vi "Waveform Test.vi"() -> (0 "error out":errorcluster, 1 "Result":bool, 2 "FileIds":string[](array[string]))   [LabVIEW 2018, in "Attach Test Files.lvlib"]
uses:
  <vilib>/Skyline/File/File/Send File.vi
  Attach Test Files.lvlib
  <vilib>/Skyline/File/File/NI Skyline File.lvclass
panel:
  out "Measured Data":dynamicdata(graph)
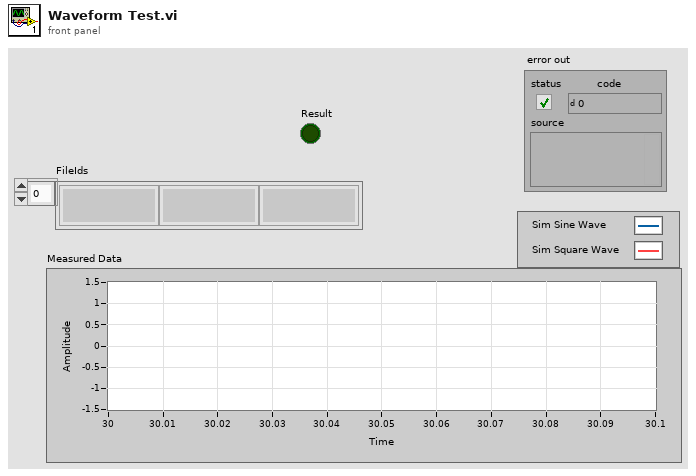
[diagram p1: front panel]
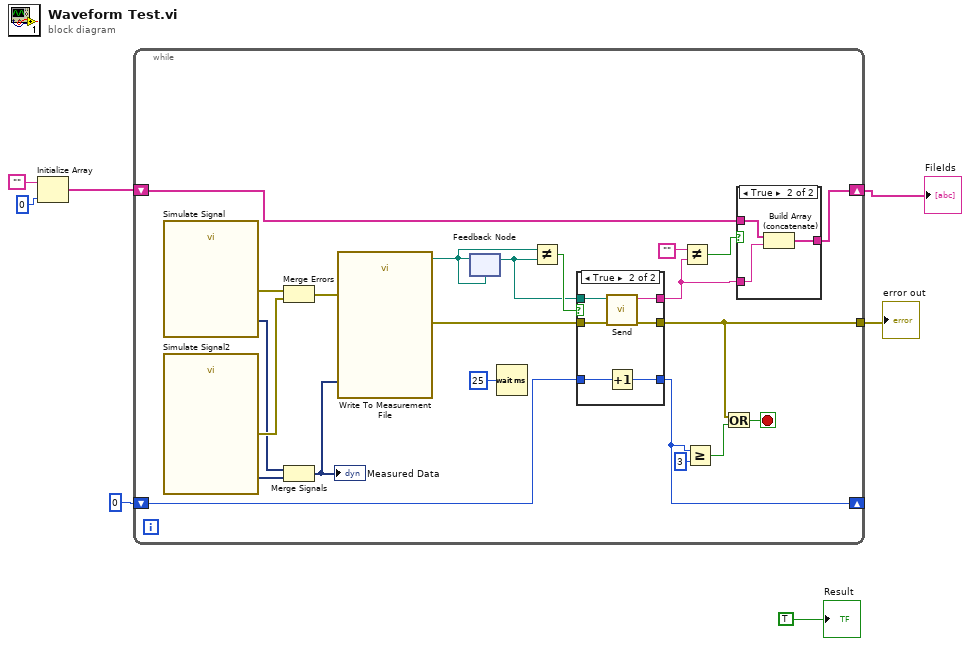
[diagram p0: block diagram]
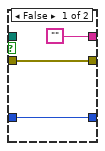
[diagram p3: hidden frame]
diagram:
  n1 = Initialize Array("", 0) -> (w4:string[])
  n2 = while {
    tunnel: [w20] -> w1
    shift-right: [w15] -> _
    shift-left: 0 -> [w16]
    shift-right: [w8] -> w2
    shift-left: w4 -> [w9]
    stop <- w24 stop-if-true
    n3 = call "Simulate Signal"() -> ("Sim Sine Wave"=w27:dynamicdata, "error out"=w29:errorcluster)  [unwired: 14 in]
    n4 = call "Simulate Signal2"() -> ("Sim Square Wave"=w26:dynamicdata, "error out"=w28:errorcluster)  [unwired: 14 in]
    n5 = Merge Errors(w29, w28) -> (w25:errorcluster)
    n6 = Merge Signals(w27, w26) -> (w22:dynamicdata)
    "Measured Data" <- w22
    n7 = call "Write To Measurement File"("Signals"=w22, "error in (no error)"=w25) -> ("Filename Out"=w17:path, "error out"=w18:errorcluster)  [unwired: 15 in, 1 out]
    n8 = feedback-in #1(w17) -> ()
    n9 = feedback #1(w17) -> (w19:path)
    n10 = Wait (ms)(milliseconds to wait=u32 25) -> ()  [unwired: 1 out]
    n11 = Not Equal?(x=w17, y=w19) -> (x != y?=w21:bool)
    n12 = case shown="True" w21 {
      tunnel: [w36 w41] -> w20
      tunnel: w19 -> [_ w40]
      tunnel: w18 -> [w36 w42]
      tunnel: w16 -> [w35 w39]
      tunnel: [w35 w38] -> w15
      tunnel: ["" w37] -> w10
      frame False {
      }
      frame True {
        n13 = call-poly <vilib>:"Send.vi"("error in (no error)"=w42, "path"=w40) -> ("error out"=w41:errorcluster, "id"=w37:string)  [unwired: 7 in]
        n14 = Increment(x=w39) -> (x+1=w38:i32)
      }
    }
    n15 = Not Equal?(x="", y=w10) -> (x != y?=w11:bool)
    n16 = Greater Or Equal?(x=w15, y=3) -> (x >= y?=w13:bool)
    n17 = Or(x=w20, y=w13) -> (x .or. y?=w24:bool)
    n18 = case shown="True" w11 {
      tunnel: w10 -> [_ w33]
      tunnel: w9 -> [w30 w32]
      tunnel: [w30 w31] -> w8
      frame False {
      }
      frame True {
        n19 = Build Array (concatenate)(w32, w33) -> (w31:string[])
      }
    }
  }
  "FileIds" <- w2
  "error out" <- w1
  "Result" <- TRUE
